vi "脉冲宽度测量实验.vi"   [LabVIEW 2011]
uses:
  <vilib>/STM32_DriverVI_Interface_F4/Timer/Filter Mode_F4.ctl
  <vilib>/STM32_DriverVI_Interface_F4/Timer/Edge Mode_F4.ctl
  <vilib>/STM32_DriverVI_Interface_F4/Timer/TIMX Interrupt_F4.ctl
  <vilib>/STM32_DriverVI_Interface_F4/Interrupt/PreemptionPriority_2_F4.ctl
  <vilib>/STM32_DriverVI_Interface_F4/Interrupt/SubPriority_2_F4.ctl
  <vilib>/STM32_DriverVI_Interface_F4/Timer/TIM5_Group_Pins_F4.ctl
  <vilib>/STM32_DriverVI_Interface_F4/Timer/TIM5_Channels_Pin_Map_F4.ctl
  <vilib>/STM32_DriverVI_Interface_F4/GPIO/GPIO_Group_Mode_Interface_F4.ctl
  <vilib>/STM32_DriverVI_Interface_F4/Timer/TIM5_Capture_Channel_F4.ctl
  <vilib>/STM32_DriverVI_Interface_F4/Timer/TIM5_Flag_F4.ctl
  <vilib>/STM32_DriverVI_Interface_F4/Timer/TIM5_Int_Channel_F4.ctl
  <vilib>/eio/EIO_TerminalDirection.ctl
  <vilib>/STM32_DriverVI_Interface_F4/Timer/TIM5 Init_F4.vi
  <vilib>/STM32_DriverVI_Interface_F4/Timer/TIM5 Channel Pin Map_F4.vi
  <vilib>/STM32_DriverVI_Interface_F4/Timer/TIM5 Channel Filter Set_F4.vi
  <vilib>/STM32_DriverVI_Interface_F4/Timer/TIM5 Channel Edge Set_F4.vi
  <vilib>/STM32_DriverVI_Interface_F4/Timer/TIM Priority Set_2_F4.vi
  <vilib>/STM32_DriverVI_Interface_F4/Timer/TIM5 SW Interrupt_F4.vi
  <vilib>/STM32_DriverVI_Interface_F4/Timer/Clear_TIM5_Flag_F4.vi
  <vilib>/STM32_DriverVI_Interface_F4/Timer/TIM5 Int Permit_UnPermit_F4.vi
  <vilib>/STM32_DriverVI_Interface_F4/Timer/TIM5 Int Enable_Disable_F4.vi
  <vilib>/STM32_DriverVI_Interface_F4/GPIO_EIO/GPO_EIO_Inner_F4.vi
  <vilib>/eio/EIONode/EIONode.xnode
types:
  T1 = typedef "TIM5_Int_Channel_F4.ctl" = enum8{"TIM5_Update(Overflow)", "TIM5_Channel_1", "TIM5_Channel_2", "TIM5_Channel_3", "TIM5_Channel_4", "TIM5_Reserved……", "TIM5_Trigger(Pulse)"}
  T2 = typedef "TIM5_Flag_F4.ctl" = enum8{"TIM5_Update(Overflow)", "TIM5_Channel_1", "TIM5_Channel_2", "TIM5_Channel_3", "TIM5_Channel_4", "TIM5_Reserved……", "TIM5_Trigger(Pulse)"}
  T3 = typedef "TIM5_Capture_Channel_F4.ctl" = enum8{"TIM5_Channel_1", "TIM5_Channel_2", "TIM5_Channel_3", "TIM5_Channel_4"}
  T4 = typedef "GPIO_Group_Mode_Interface_F4.ctl" = enum8{"Floating Input", "Pull-up Input", "Pull-down Input", "-----------------------", "Push-pull Output", "Open-drain Output"}[]
  T5 = typedef "TIM5_Group_Pins_F4.ctl" = T6[]
  T6 = typedef "TIM5_Channels_Pin_Map_F4.ctl" = enum8{"TIM5_Channel_1-->PA0", "TIM5_Channel_1-->PH10", "TIM5_Channel_2-->PA1", "TIM5_Channel_2-->PH11", "TIM5_Channel_3-->PA2", "TIM5_Channel_3-->PH12", "TIM5_Channel_4-->PA3", "TIM5_Channel_4-->PI0"}
  T7 = typedef "中断使能禁止.ctl" = enum8{"Disable", "Enable"}
  T8 = typedef "允许或禁止TIM中断_F4.ctl" = enum8{"禁止", "允许"}
  T9 = typedef "SubPriority_2_F4.ctl" = enum8{"Priority_0（High）", "Priority_1", "Priority_2", "Priority_3（Low）"}
  T10 = typedef "PreemptionPriority_2_F4.ctl" = enum8{"Priority_0（Highest）", "Priority_1", "Priority_2", "Priority_3（Lowest）"}
  T11 = typedef "TIMX Interrupt_F4.ctl" = u8
  T12 = typedef "Edge Mode_F4.ctl" = enum8{"Rising edge", "Falling edge"}
  T13 = typedef "Filter Mode_F4.ctl" = enum8{"None Filter", "2 Points Filter", "4 Points Filter", "8 Points Filter"}
  T14 = typedef "TIMX计数时钟频率_F4.ctl" = u16
  T15 = enum8{"P0", "P1", "P2", "P3", "P4", "P5", "P6", "P7", "P8", "P9", "P10", "P11", "P12", "P13", "P14", "P15"}
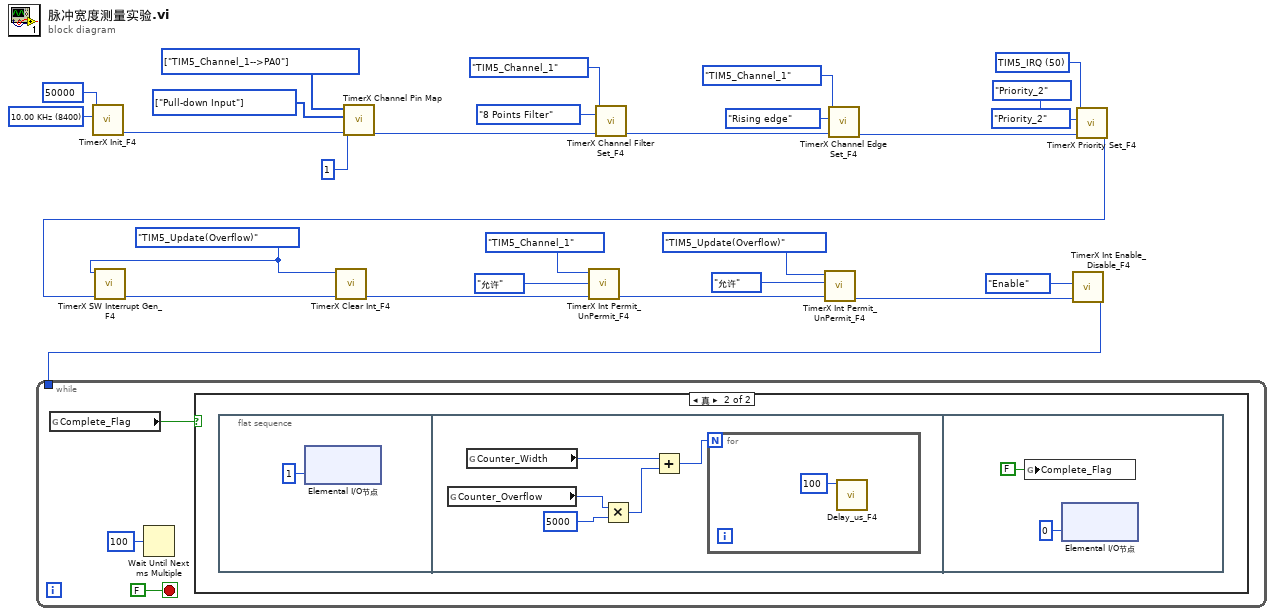
[diagram p0: block diagram]
diagram:
  w5 = TIM5_Flag_F4."TIM5_Update(Overflow)" ("TIM5_Flag")
  w2 = T4 [enum."Pull-down Input"] items=["Floating Input", "Pull-up Input", "Pull-down Input", "-----------------------", "Push-pull Output", "Open-drain Output"] ("GPIO Mode Set")
  w8 = T5 [enum."TIM5_Channel_1-->PA0"] items=["TIM5_Channel_1-->PA0", "TIM5_Channel_1-->PH10", "TIM5_Channel_2-->PA1", "TIM5_Channel_2-->PH11", "TIM5_Channel_3-->PA2", "TIM5_Channel_3-->PH12", "TIM5_Channel_4-->PA3", "TIM5_Channel_4-->PI0"] ("TIM5 Group Channel Pins")
  w20 = T11 50 items=["WWDG_IRQ"=0, "RTC_WKUP_IRQ"=3, "RTC_Alarm_IRQ"=41, "TIM1_BRK_TIM9_IRQ"=24, "TIM1_UP_TIM10_IRQ"=25, "TIM1_TRG_COM_TIM11_IRQ"=26, "TIM1_CC_IRQ"=27, "TIM2_IRQ"=28, "TIM3_IRQ"=29, "TIM4_IRQ"=30, "TIM5_IRQ"=50, "TIM6_IRQ"=54, "TIM7_IRQ"=55, "TIM8_BRK_TIM12_IRQ"=43, "TIM8_UP_TIM13_IRQ"=44, "TIM8_TRG_COM_TIM14_IRQ"=45, "TIM8_CC_IRQ"=46] ("TIM 中断号设置")
  w27 = T14 8400 items=["84.00 MHz"=1, "42.00 MHz"=2, "28.00 MHz"=3, "21.00 MHz"=4, "12.000 MHz"=7, "7.000 MHz"=12, "4.000 MHz"=21, "1.000 MHz"=84, "-------------"=0, "500.0 KHz"=168, "250.0 KHz"=336, "100.0 KHz"=840, "50.00 KHz"=1680, "10.00 KHz"=8400] ("时钟预分频数")
  n1 = call-poly <vilib>:"TimerX Init_F4.vi"("时钟预分频数"=w27, "自动重装值"=u16 50000) -> ("err_out"=w26:u8)  [unwired: 9 in]
  n2 = call-poly <vilib>:"TimerX Channel Pin Map.vi"("err_in"=w26, "Group_Length"=u8 1, "GPIO Mode Set"=w2, "TIM5 Group Channel Pins"=w8) -> ("err_out"=w25:u8)  [unwired: 7 in]
  n3 = call-poly <vilib>:"TimerX Channel Filter Set_F4.vi"("err_in"=w25, "Filter Mode"=Filter_Mode_F4."8 Points Filter", "TIM5_Capture_Channel"=TIM5_Capture_Channel_F4."TIM5_Channel_1") -> ("err_out"=w23:u8)  [unwired: 8 in]
  n4 = call-poly <vilib>:"TimerX Channel Edge Set_F4.vi"("err_in"=w23, "Edge Mode"=Edge_Mode_F4."Rising edge", "TIM5_Capture_Channel"=TIM5_Capture_Channel_F4."TIM5_Channel_1") -> ("err_out"=w21:u8)  [unwired: 8 in]
  n5 = call-poly <vilib>:"TimerX Priority Set_F4.vi"("err_in"=w21, "响应优先级"=SubPriority_2_F4."Priority_2", "抢占优先级"=PreemptionPriority_2_F4."Priority_2", "IO 中断号设置"=w20) -> ("err_out"=w17:u8)  [unwired: 6 in, 1 out]
  n6 = call-poly <vilib>:"TimerX SW Interrupt Gen_F4.vi"("err_in"=w17, "TIM5_Flag"=w5) -> ("err_out"=w16:u8)  [unwired: 9 in]
  n7 = call-poly <vilib>:"TimerX Clear Int_F4.vi"("err_in"=w16, "TIM5_Flag"=w5) -> ("err_out"=w15:u8)  [unwired: 9 in]
  n8 = call-poly <vilib>:"TimerX Int Permit_UnPermit_F4.vi"("err_in"=w15, "屏蔽或开启TIM4中断"=允许或禁止TIM中断_F4."允许" ("屏蔽或开启TIM2中断"), "TIM5_Int_Channel"=TIM5_Int_Channel_F4."TIM5_Channel_1") -> ("err_out"=w13:u8)  [unwired: 8 in]
  n9 = call-poly <vilib>:"TimerX Int Permit_UnPermit_F4.vi"("err_in"=w13, "屏蔽或开启TIM4中断"=允许或禁止TIM中断_F4."允许" ("屏蔽或开启TIM2中断"), "TIM5_Int_Channel"=TIM5_Int_Channel_F4."TIM5_Update(Overflow)") -> ("err_out"=w12:u8)  [unwired: 8 in]
  n10 = call-poly <vilib>:"TimerX Int Enable_Disable_F4.vi"("err_in"=w12, "中断使能/关闭"=中断使能禁止."Enable") -> ("err_out"=w9:u8)  [unwired: 9 in]
  n11 = while {
    tunnel: w9 -> [_]
    stop <- FALSE stop-if-true
    n12 = global read "全局变量.vi" "Complete_Flag"() -> (w29:bool)
    n13 = Wait Until Next ms Multiple(millisecond multiple=u32 100 ("毫秒倍数")) -> ()  [unwired: 1 out]
    n14 = case shown="真" w29 {
      frame False {
      }
      frame True {
        n15 = flat-sequence {
          frame #0 {
            n16 = xnode "Elemental I/O节点"("BEEP"=u8 1) -> ()  [unwired: 1 in, 1 out]
          }
          frame #1 {
            n17 = global read "全局变量.vi" "Counter_Overflow"() -> (w41:i32)
            n18 = global read "全局变量.vi" "Counter_Width"() -> (w38:i32)
            n19 = Multiply(x=w41, y=5000) -> (x*y=w39:i32)
            n20 = Add(x=w38, y=w39) -> (x+y=w37:i32)
            n21 = for {
              N: w37 -> [_]
              n22 = call <vilib>:"Delay_us_F4.vi"("time_us（1~798915）"=u32 100) -> ()  [unwired: 10 in, 1 out]
            }
          }
          frame #2 {
            n23 = global write "全局变量.vi" "Complete_Flag"(FALSE ("Complete_Flag")) -> ()
            n24 = xnode "Elemental I/O节点"("BEEP"=u8 0) -> ()  [unwired: 1 in, 1 out]
          }
        }
      }
    }
  }
